vi "FormatConditional.vi"(4 "else":string[](array[string]), 5 "if":string[](array[string]), 9 "condition":string) -> (3 "python":string)   [LabVIEW 2014, in "Python Functions.lvlib"]
uses:
  Python Functions.lvlib
  <vilib>/Utility/error.llb/whitespace.ctl
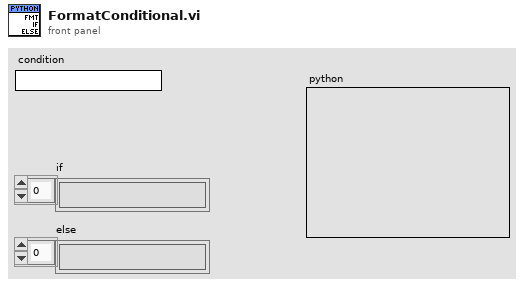
[diagram p1: front panel]
types:
  T1 = typedef "whitespace.ctl" = u16
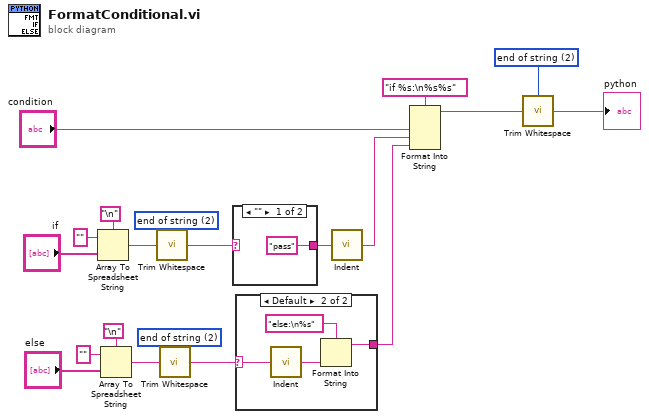
[diagram p0: block diagram]
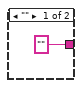
[diagram p2: hidden frame]
diagram:
  w7 = T1 2 items=["both", "start of string", "end of string"] ("location (both)")
  w10 = T1 2 items=["both", "start of string", "end of string"] ("location (both)")
  w16 = T1 2 items=["both", "start of string", "end of string"] ("location (both)")
  n1 = Array To Spreadsheet String(delimiter (Tab)="\n", array="if", 3:"" ("format string")) -> (spreadsheet string=w17:string)
  n2 = Array To Spreadsheet String(delimiter (Tab)="\n", array="else", 3:"" ("format string")) -> (spreadsheet string=w6:string)
  n3 = call <vilib>:"Trim Whitespace.vi"("string"=w17, "location (both)"=w16) -> ("trimmed string"=w15:string)
  n4 = call <vilib>:"Trim Whitespace.vi"("string"=w6, "location (both)"=w7) -> ("trimmed string"=w8:string)
  n5 = case shown="\"\"" w15 {
    selector: w15 -> [_ w22]
    tunnel: ["pass" w22] -> w14
    frame "" {
    }
    frame Default {
    }
  }
  n6 = case shown="Default" w8 {
    selector: w8 -> [_ w27]
    tunnel: ["" w24] -> w1
    frame "" {
    }
    frame Default {
      n7 = call "Indent.vi"("string in"=w27) -> ("string out"=w26:string)  [unwired: 1 in]
      n8 = Format Into String(format string="else:\n%s", w26) -> (resulting string=w24:string)  [unwired: 2 in, 1 out]
    }
  }
  n9 = call "Indent.vi"("string in"=w14) -> ("string out"=w2:string)  [unwired: 1 in]
  n10 = Format Into String(format string="if %s:\n%s%s", "condition", w2, w1) -> (resulting string=w12:string)  [unwired: 2 in, 1 out]
  n11 = call <vilib>:"Trim Whitespace.vi"("string"=w12, "location (both)"=w10) -> ("trimmed string"=→"python":string)
